vi "testBothPDs.vi"() -> ()   [LabVIEW 2018]
panel:
  in  "stop":bool
  out "error out 2":errorcluster caption="error out"
  out "error out":errorcluster
  out "Power 2":dbl format="%_7g"
  out "Power":dbl format="%_7g"
  out "Transmittance PD 1/2":dbl
  out "Initialized PD 2":bool
  out "Initialized PD":bool
  in  "resource name 2":refnum<visa-resource-name> caption="resource name"
  in  "resource name":refnum<visa-resource-name>
  # "EL PD1 Es el larguito (51 INSTR), el PD2 es el naranja esferico (53 INSTR)"
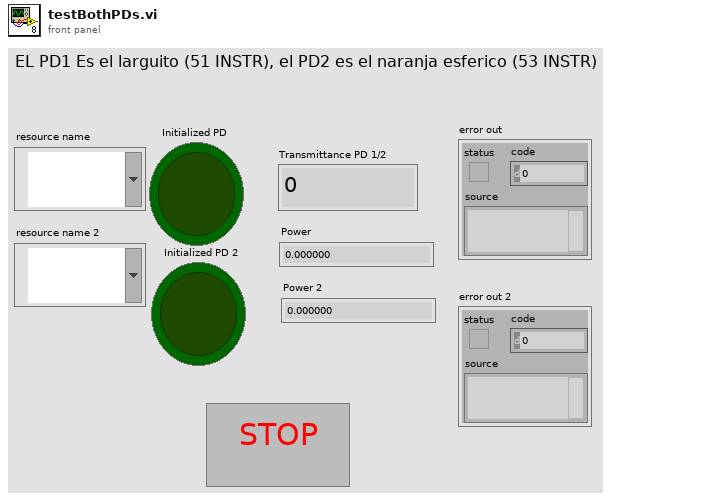
[diagram p1: front panel]
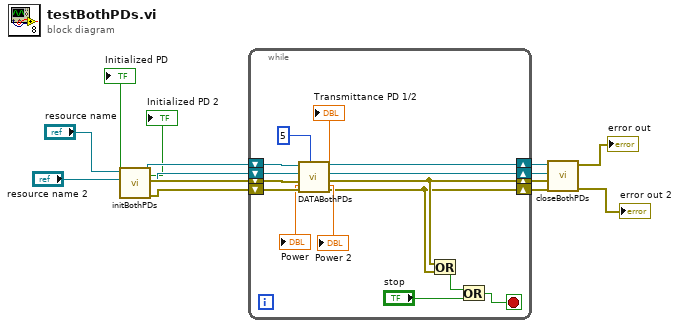
[diagram p0: block diagram]
diagram:
  n1 = call "initBothPDs.vi"("resource name 2"="resource name 2", "resource name"="resource name") -> ("error IO 2"=w9:errorcluster, "error IO"=w12:errorcluster, "instrument handle out 2"=w8:refnum<visa-resource-name>, "instrument handle out"=w13:refnum<visa-resource-name>, "Initialized PD"=→"Initialized PD" →"Initialized PD 2":bool)  [unwired: 4 in, 1 out]
  n2 = while {
    shift-right: [w26] -> w11
    shift-left: w13 -> [w28]
    shift-right: [w18] -> w10
    shift-left: w12 -> [w27]
    shift-right: [w17] -> w6
    shift-left: w9 -> [w25]
    shift-right: [w23] -> w7
    shift-left: w8 -> [w24]
    stop <- w14 stop-if-true
    n3 = call "DATABothPDs.vi"("loops x measure"=5, "error in 2"=w25, "error in 1"=w27, "Visa Ref in 2"=w24, "Visa Ref in 1"=w28) -> ("error out 2"=w17:errorcluster, "error out 1"=w18:errorcluster, "Visa ref out2"=w23:refnum<visa-resource-name>, "Visa ref out 1"=w26:refnum<visa-resource-name>, "Power 2"=→"Power 2":dbl, "Transmittance PD 1/2"=→"Transmittance PD 1/2":dbl, "Power"=→"Power":dbl)
    n4 = Or(x=w18, y=w17) -> (x .or. y?=w16:bool)
    n5 = Or(x=w16, y="stop") -> (x .or. y?=w14:bool)
  }
  n6 = call "closeBothPDs.vi"("error in (no error) 2"=w6, "error in (no error)"=w10, "instrument handle 2"=w7, "instrument handle"=w11) -> ("error out 2"=→"error out 2":errorcluster, "error out"=→"error out":errorcluster)  [unwired: 6 in]
